vi "Manual.vi"(6 "Cluster":T12={"VISA resource name"="", "baud rate "=115200}, 7 "vi reference":refnum<vi>, 8 "error in (no error)":errorcluster, 9 "IOList_280":T1, 11 "Manual":T4(tab)) -> (0 "error out":errorcluster, 3 "Out reference":refnum<vi>)   [LabVIEW 2015]
uses:
  Control Button/Exit.ctl
  Control Button/Scanner config.ctl
  Control Button/Save.ctl
  Galobal variable_TI.vi
  <vilib>/addons/database/Connection.llb/DB Tools Open Connec (String).vi
  <vilib>/Instr/_visa.llb/VISA Configure Serial Port (Instr).vi
  <vilib>/addons/database/_DB Variant To Data/Database Variant To Data.xnode
  <vilib>/addons/database/NI_Database_API.lvlib
panel:
  out "Array":string[](array[string])
  out "Byte Lenth":i32
  out "error out 2":errorcluster
  in  "Stop":T2
  out "NewVal":T3
  in  "Digital Output":T5
  out "LVDT":string
  out "Digital Input":T6
  in  "Trigger For Model":bool
  in  "Program List":string(combo)
  in  "Home Calling M1":bool
  in  "Stop M1":bool
  in  "SERVO ON CMD M1":bool
  in  "Speed (mm/s) M1":i32=10
  in  "Travel (mm)M1":i32=5
  out "STM1 Done Bit":bool
  out "Error Message":string
  in  "Save":T7
  in  "Sensor Setting Data":T8 {"IL Sensor_Max (AI12)" format="%0.02f"; "IL Sensor_Max (AI11)" format="%0.02f"; "IL Sensor_Max (AI10)" format="%0.02f"; "IL Sensor_Max (AI9)" format="%0.02f"; "IL Sensor1_Max AI1" format="%0.02f"; "IL Sensor1_Max AI0" format="%0.02f"; "IL Sensor_Min (AI12" format="%0.02f"; "IL Sensor_Min (AI11)" format="%0.02f"; "IL Sensor_Min(AI10)" format="%0.02f"; "IL Sensor_Min  (AI9)" format="%0.02f"; "IL Sensor1_ Min AI1" format="%0.02f"; "IL Sensor1_Min AI0" format="%0.02f"}
  out "Sensor Data":T9 {"IL Sensor  (AI12" format="%0.02f"; "IL Sensor (AI11)" format="%0.02f"; "IL Sensor  (AI10)" format="%0.02f"; "IL Sensor (AI9)" format="%0.02f"; "IL Sensor1_AI1" format="%0.02f"; "IL Sensor1_AI0" format="%0.02f"}
  in  "Barcode Trigger":T10(ring)
  out "Error Status":bool
  in  "Scanner config":T11
  out "Read data":string
  out "Boolean":bool
  # "Instruction for Servo motor Operate\n(1)  Switch  ON -OFF  of Fixture Slide servo Brake ON Cmd (P0.19)  \n      from Digital Output tab.\n(2) Switch  ON -OFF  of Fixture Slide Servo Direction Command (P0.20)\n      from Digital Output tab."
  # "Fixture Slide servo"
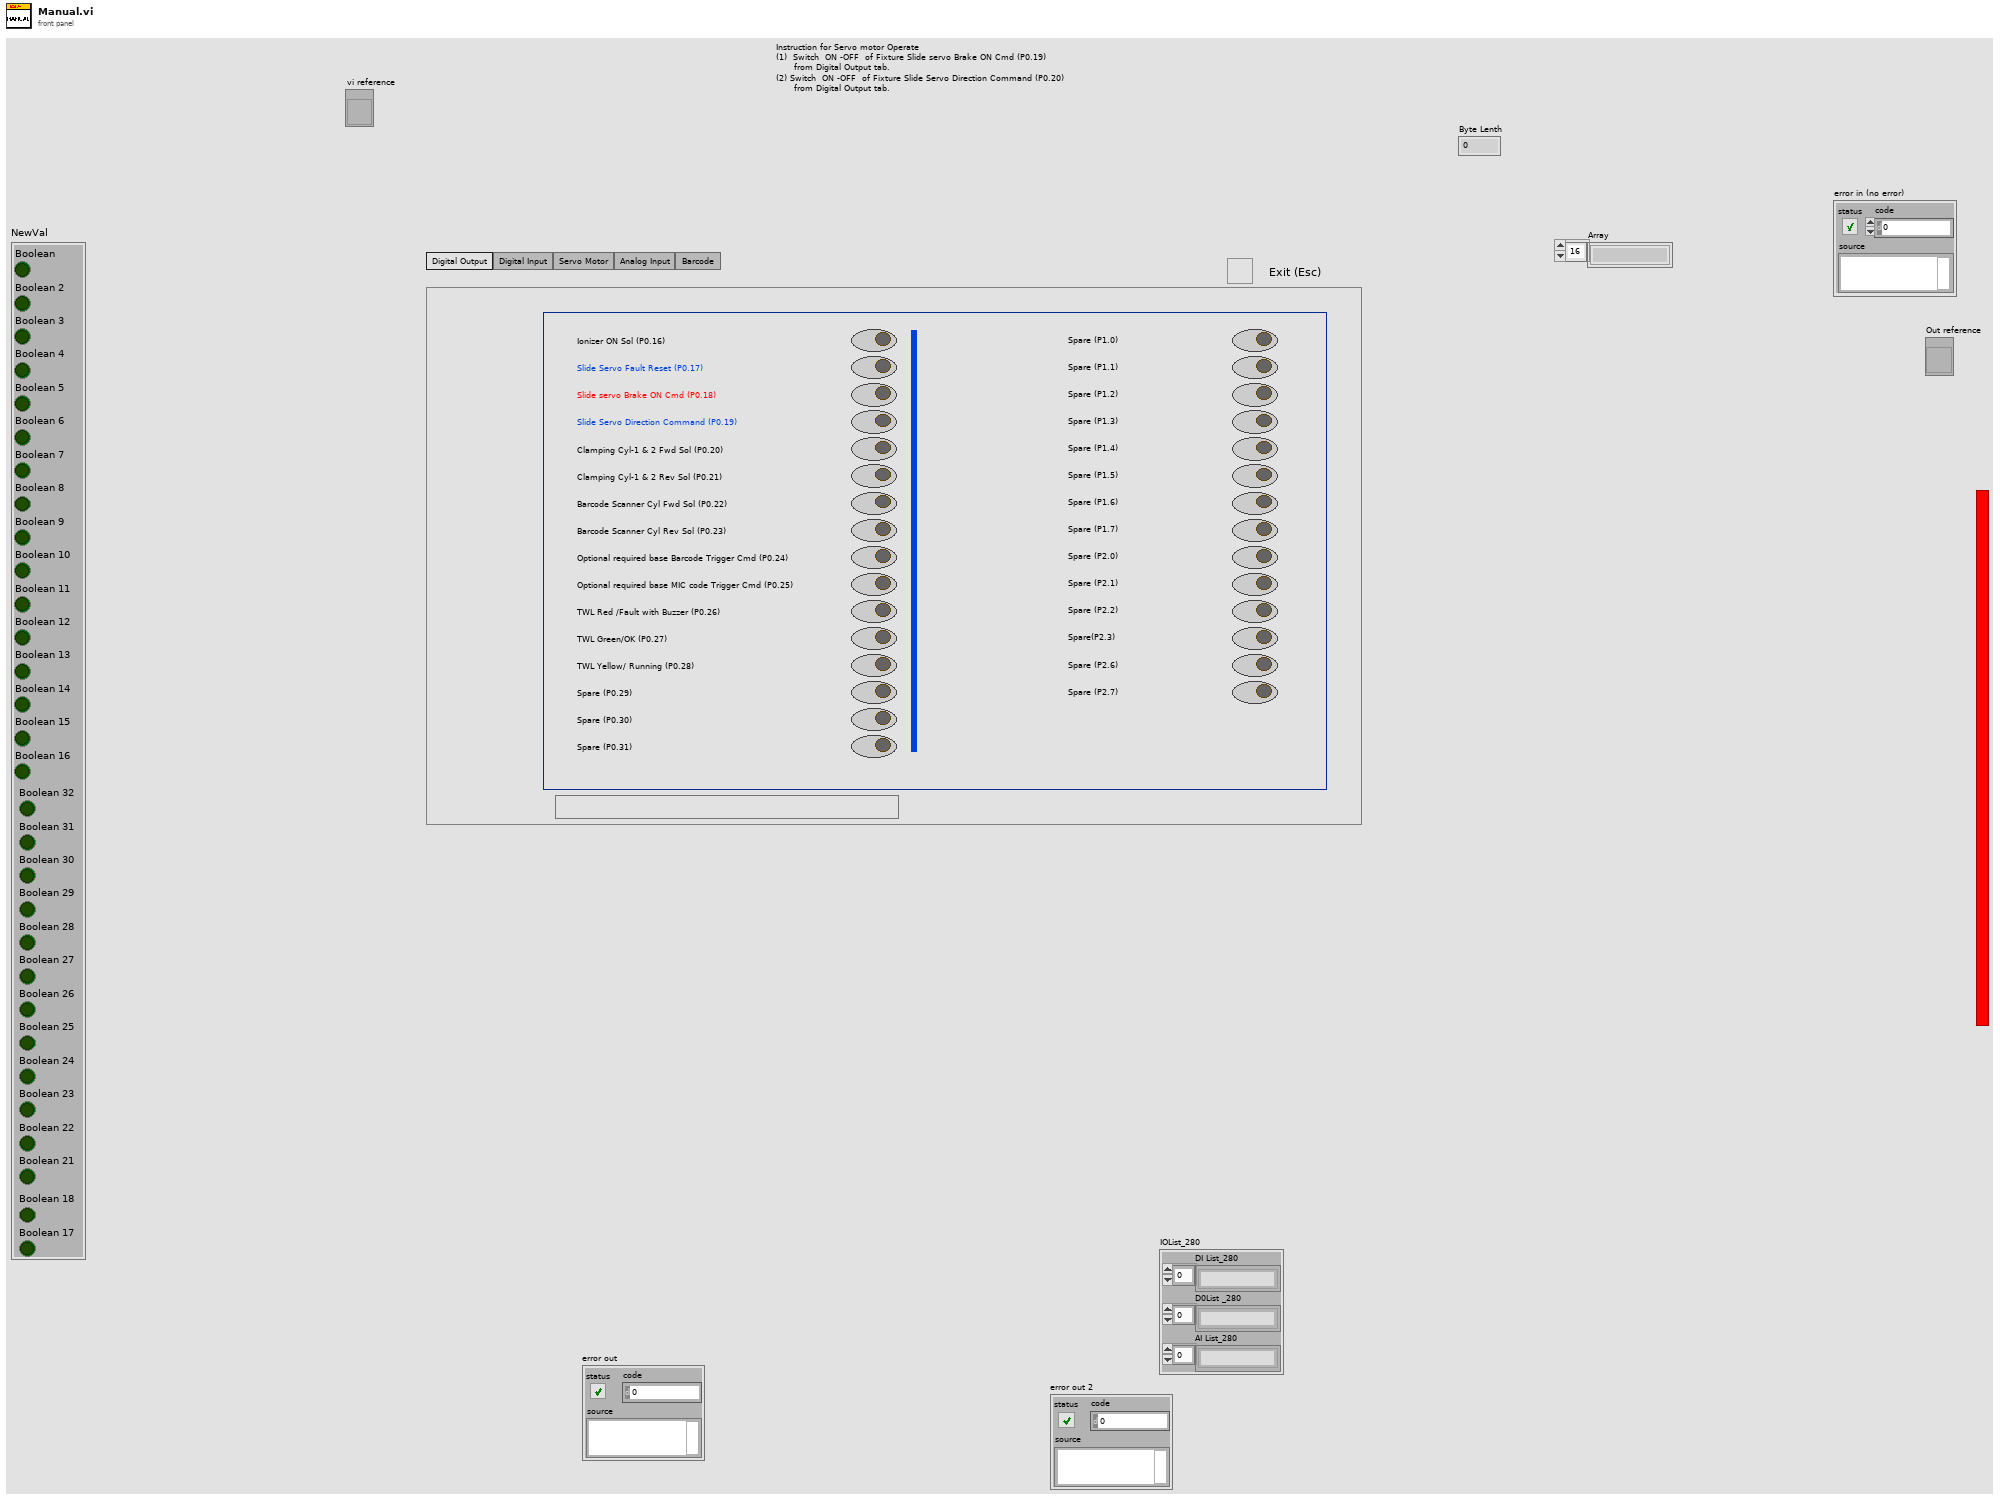
[diagram p1: front panel]
types:
  T1 = cluster{"DI List_280":string[], "D0List _280":string[], "AI List_280":string[]}
  T2 = typedef "Exit.ctl" = bool
  T3 = cluster{"Boolean":bool, "Boolean 2":bool, "Boolean 3":bool, "Boolean 4":bool, "Boolean 5":bool, "Boolean 6":bool, "Boolean 7":bool, "Boolean 8":bool, "Boolean 9":bool, "Boolean 10":bool, "Boolean 11":bool, "Boolean 12":bool, "Boolean 13":bool, "Boolean 14":bool, "Boolean 15":bool, "Boolean 16":bool, "Boolean 17":bool, "Boolean 18":bool, "Boolean 21":bool, "Boolean 22":bool, "Boolean 23":bool, "Boolean 24":bool, "Boolean 25":bool, "Boolean 26":bool, "Boolean 27":bool, "Boolean 28":bool, "Boolean 29":bool, "Boolean 30":bool, "Boolean 31":bool, "Boolean 32":bool}
  T4 = enum32{"Digital Output", "Digital Input", "Servo Motor ", "Analog Input", "Barcode "}
  T5 = cluster{"DO.00":bool, "DO.01":bool, "DO.02":bool, "DO.03":bool, "DO.04":bool, "DO.05":bool, "DO.06":bool, "DO.06":bool, "DO.07":bool, "DO.08":bool, "DO.09":bool, "DO.10":bool, "DO.11":bool, "DO.12":bool, "DO.13":bool, "DO.14":bool, "DO.07 2":bool, "DO.08 2":bool, "DO.09 2":bool, "DO.10 2":bool, "DO.11 2":bool, "DO.12 2":bool, "DO.13 2":bool, "DO.14 2":bool, "DO.00 2":bool, "DO.01 2":bool, "DO.02 2":bool, "DO.03 2":bool, "DO.06 2":bool, "DO.06 3":bool}
  T6 = cluster{"Digital Input":bool, "Digital Input 2":bool, "Digital Input 3":bool, "Digital Input 4":bool, "Digital Input 5":bool, "Digital Input 6":bool, "Digital Input 7":bool, "Digital Input 8":bool, "Digital Input 9":bool, "Digital Input 10":bool, "Digital Input 11":bool, "Digital Input 12":bool, "Digital Input 13":bool, "Digital Input 14":bool, "Digital Input 15":bool, "Digital Input 16":bool, "Digital Input 17":bool, "Digital Input 18":bool, "Digital Input 19":bool, "Digital Input 20":bool, "Digital Input 21":bool, "Digital Input 22":bool, "Digital Input 23":bool, "Digital Input 24":bool, "Digital Input 25":bool, "Digital Input 26":bool, "Digital Input 27":bool, "Digital Input 28":bool, "Digital Input 29":bool, "Digital Input 30":bool, "Digital Input 31":bool, "Digital Input 32":bool, "Digital Input 33":bool, "Digital Input 34":bool, "Digital Input 35":bool, "Digital Input 36":bool, "Digital Input 37":bool, "Digital Input 38":bool, "Digital Input 39":bool, "Digital Input 40":bool, "Digital Input 41":bool, "Digital Input 42":bool, "Digital Input 43":bool, "Digital Input 44":bool}
  T7 = typedef "Save.ctl" = bool
  T8 = cluster{"IL Sensor1_Max AI0":dbl, "IL Sensor1_Min AI0":dbl, "IL Sensor1_Max AI1":dbl, "IL Sensor1_ Min AI1":dbl, "IL Sensor_Max (AI9)":dbl, "IL Sensor_Min  (AI9)":dbl, "IL Sensor_Max (AI10)":dbl, "IL Sensor_Min(AI10)":dbl, "IL Sensor_Max (AI11)":dbl, "IL Sensor_Min (AI11)":dbl, "IL Sensor_Max (AI12)":dbl, "IL Sensor_Min (AI12":dbl}
  T9 = cluster{"IL Sensor1_AI0":dbl, "IL Sensor1_AI1":dbl, "IL Sensor (AI9)":dbl, "IL Sensor  (AI10)":dbl, "IL Sensor (AI11)":dbl, "IL Sensor  (AI12":dbl, "IL Sensor1_AI0":bool, "IL Sensor1_AI1":bool, "IL Sensor1_AI9":bool, "IL Sensor1_AI10":bool, "IL Sensor1_AI11":bool, "IL Sensor1_AI12":bool}
  T10 = enum16{"LCD BArcode Trigger", "MIC Barcode Trigger"}
  T11 = typedef "Scanner config.ctl" = bool
  T12 = cluster{"VISA resource name":refnum<visa-resource-name>, "baud rate ":u32}
  T13 = typedef "NI_Database_API.lvlib/Conn ObjectReference.ctl" = refnum<k1>
  T14 = cluster{" Fixture Brack on":refnum<vi>, " Fixture Direction":refnum<vi>, "Servo Cmd":refnum<vi>, "Servo Home":refnum<vi>}
  T15 = cluster{"Emergency_1":bool, "Reset_2":bool, "Air Pressure_4":bool, "Safety Sensor_5":bool, "Safety Sensor_6":bool, "Barcode Rev rs_24":bool, "Clamp fwd rs_21":bool, "Servo Fault":bool, "Home _3":bool}
  T16 = cluster{"IL Sensor1_AI0":dbl, "IL Sensor1_AI1":dbl, "IL Sensor (AI6)":dbl, "IL Sensor  (AI7)":dbl, "IL Sensor (AI8)":dbl, "IL Sensor  (AI9)":dbl, "IL Sensor1_AI0":bool, "IL Sensor1_AI1":bool, "IL Sensor1_AI9":bool, "IL Sensor1_AI10":bool, "IL Sensor1_AI11":bool, "IL Sensor1_AI12":bool}
  T17 = cluster{"Digital input[0]":bool, "Digital input[1]":bool, "Digital input[2]":bool, "Digital input[3]":bool, "Digital input[4]":bool, "Digital input[5]":bool, "Digital input[6]":bool, "Digital input[7]":bool, "Digital input[8]":bool, "Digital input[9]":bool, "Digital input[10]":bool, "Digital input[11]":bool, "Digital input[12]":bool, "Digital input[13]":bool, "Digital input[14]":bool, "Digital input[15]":bool, "Digital input[16]":bool, "Digital input[17]":bool, "Digital input[18]":bool, "Digital input[19]":bool, "Digital input[20]":bool, "Digital input[21]":bool, "Digital input[22]":bool, "Digital input[23]":bool, "Digital input[24]":bool, "Digital input[25]":bool, "Digital input[26]":bool, "Digital input[27]":bool, "Digital input[28]":bool, "Digital input[29]":bool, "Digital input[30]":bool, "Digital input[31]":bool, "Digital input[32]":bool, "Digital input[33]":bool, "Digital input[34]":bool, "Digital input[35]":bool, "Digital input[36]":bool, "Digital input[37]":bool, "Digital input[38]":bool, "Digital input[39]":bool, "Digital input[40]":bool, "Digital input[41]":bool, "Digital input[42]":bool, "Digital input[43]":bool}
  T18 = cluster{"IL Sensor1_Max AI0":dbl, "IL Sensor1_Min AI0":dbl, "IL Sensor1_Max AI1":dbl, "IL Sensor1_ Min AI1":dbl, "IL Sensor_Max (AI9)":dbl, "IL Sensor_Min  (AI9)":dbl, "IL Sensor_Max (AI10)":dbl, "IL Sensor_Min(AI10)":dbl, "IL Sensor_Max (AI11)":dbl, "IL Sensor_Min (AI11)":dbl, "IL Sensor_Max (AI12)":dbl, "IL Sensor_Min (AI12":dbl, "Key":string}
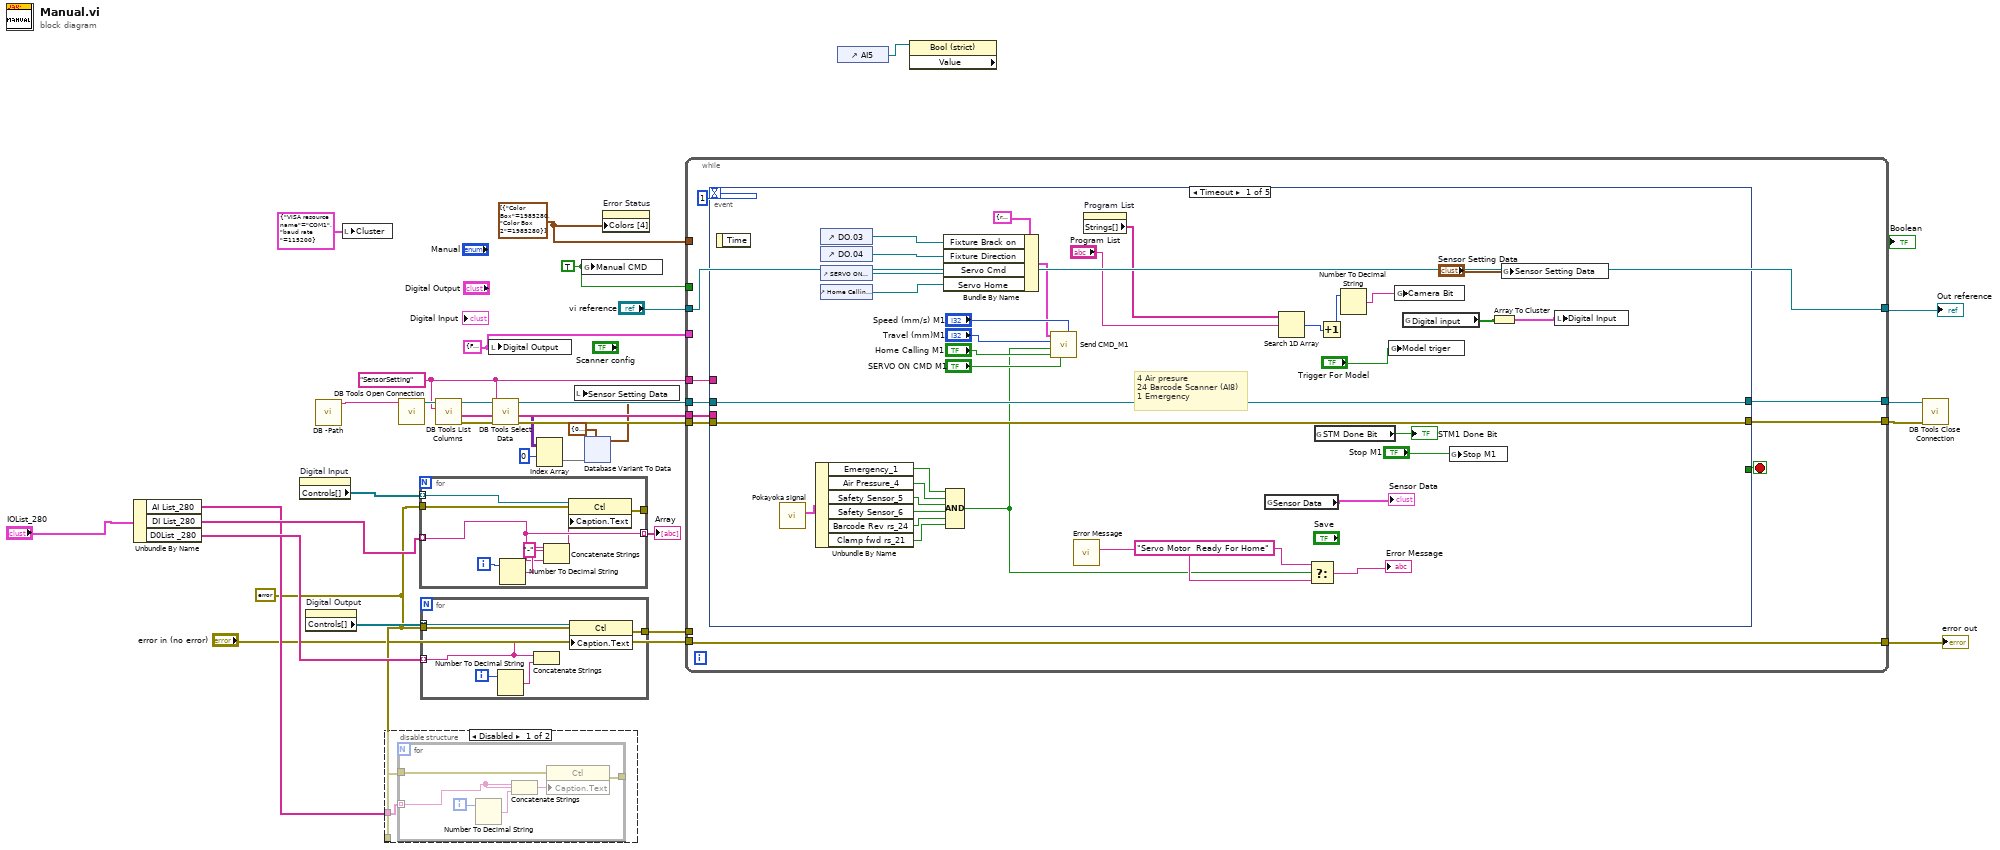
[diagram p0: block diagram]
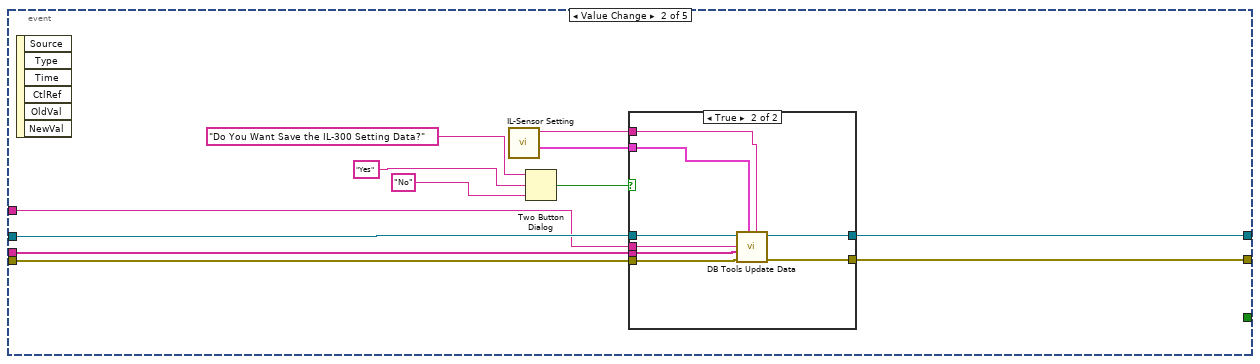
[diagram p3: hidden frame]
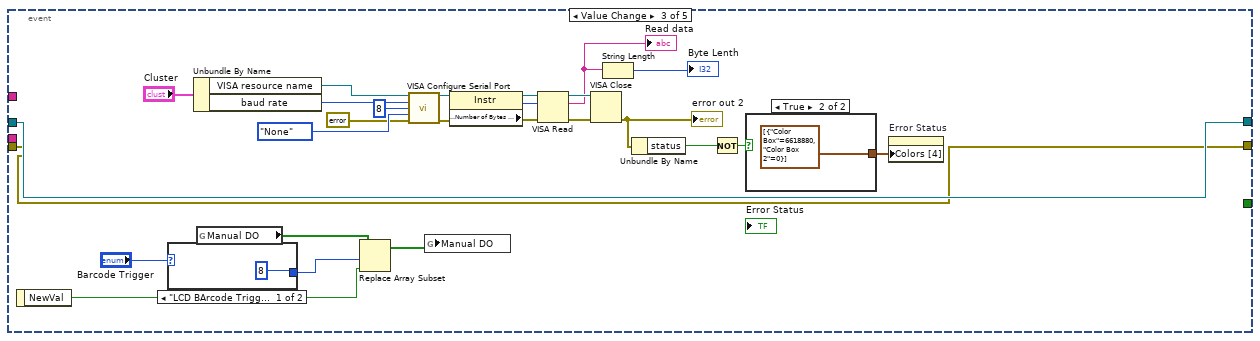
[diagram p5: hidden frame]
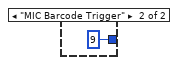
[diagram p6: hidden frame]
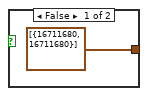
[diagram p7: hidden frame]
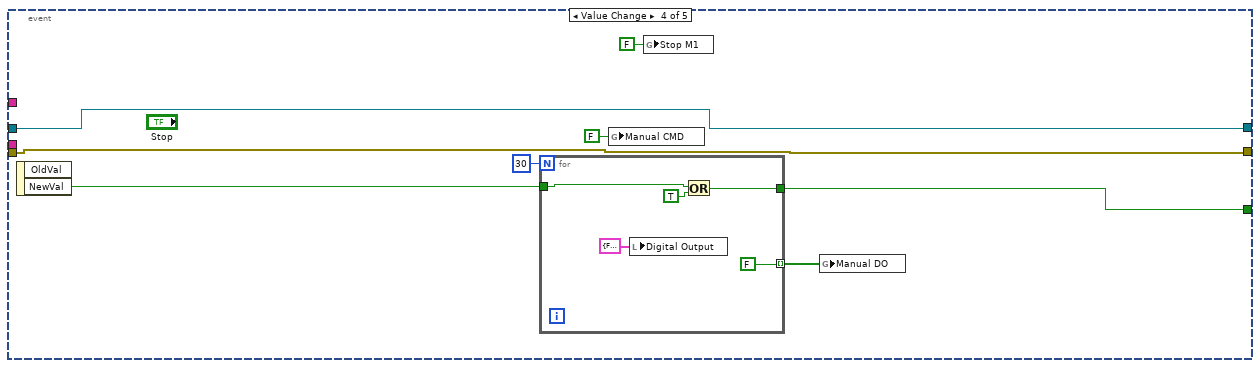
[diagram p8: hidden frame]
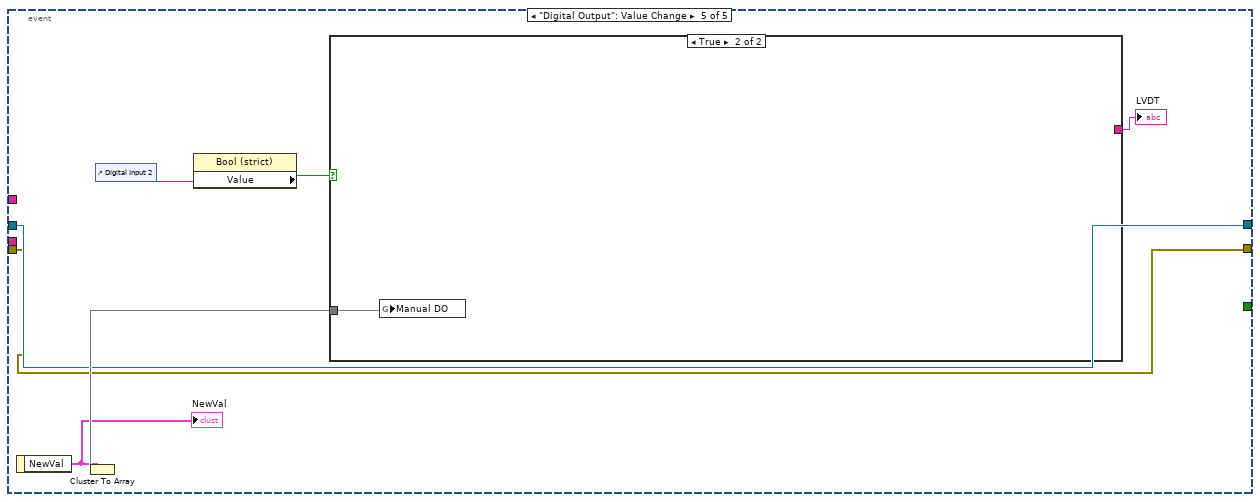
[diagram p9: hidden frame]
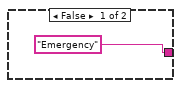
[diagram p10: hidden frame]
diagram:
  w11 = "SensorSetting" ("table")
  w18 = T5 {"DO.00"=FALSE, "DO.01"=FALSE, "DO.02"=FALSE, "DO.03"=FALSE, "DO.04"=FALSE, "DO.05"=FALSE, "DO.06"=FALSE, "DO.06"=FALSE, "DO.07"=FALSE, "DO.08"=FALSE, "DO.09"=FALSE, "DO.10"=FALSE, "DO.11"=FALSE, "DO.12"=FALSE, "DO.13"=FALSE, "DO.14"=FALSE, "DO.07 2"=FALSE, "DO.08 2"=FALSE, "DO.09 2"=FALSE, "DO.10 2"=FALSE, "DO.11 2"=FALSE, "DO.12 2"=FALSE, "DO.13 2"=FALSE, "DO.14 2"=FALSE, "DO.00 2"=FALSE, "DO.01 2"=FALSE, "DO.02 2"=FALSE, "DO.03 2"=FALSE, "DO.06 2"=FALSE, "DO.06 3"=FALSE} ("Digital Output")
  w21 = errorcluster {"status"=FALSE, "code"=0, "source"=""} ("error in (no error)")
  w24 = cluster{"Color Box":u32, "Color Box 2":u32}[] [{"Color Box"=1985280, "Color Box 2"=1985280}] ("Colors [4]")
  w29 = TRUE ("Manual CMD")
  n1 = Unbundle By Name("IOList_280") -> ("AI List_280"=w25:string[], "DI List_280"=w26:string[], "D0List _280"=w28:string[])
  n2 = property on="Digital Input" class="Clust (strict)"() -> ("Controls[]"=w27:refnum<vi>[])  [unwired: 2 in, 2 out]
  n3 = property on="Digital Output" class="Clust (strict)"() -> ("Controls[]"=w32:refnum<vi>[])  [unwired: 2 in, 2 out]
  n4 = call "DB -Path.vi"() -> ("String"=w15:string)  [unwired: 11 in]
  n5 = local write "Cluster"(T12 {"VISA resource name"="COM1", "baud rate "=115200} ("Cluster")) -> ()
  n6 = disable-structure shown="Disabled" {
    disable-tunnel: w25 -> [w35 _]
    disable-tunnel: w21 -> [w34 _]
    frame Disabled {
      n7 = for {
        tunnel: [w39] -> _
        tunnel: w34 -> [w37]
        tunnel: w35 -> [w36] mode=indexing
        i -> [w40]
        n8 = Number To Decimal String(number=w40) -> (decimal integer string=w38:string)  [unwired: 1 in]
        n9 = Concatenate Strings(w36, w38) -> ()  [unwired: 1 out]
        n10 = property class="Ctl"(error in=w37, "Caption.Text"=w36) -> (error out=w39:errorcluster)  [unwired: 1 in, 1 out]
      }
    }
    frame Enabled {
    }
  }
  n11 = call-poly <vilib>:"DB Tools Open Connection.vi"("connection information"=w15) -> ("connection reference"=w16:T13)  [unwired: 7 in, 1 out]
  n12 = for {
    tunnel: w27 -> [w48] mode=indexing
    tunnel: [w46] -> _
    tunnel: w21 -> [w45]
    tunnel: w26 -> [w42] mode=indexing
    tunnel: [w42] -> w22 mode=indexing
    i -> [w47]
    n13 = Number To Decimal String(number=w47) -> (decimal integer string=w44:string)  [unwired: 1 in]
    n14 = Concatenate Strings(w44, "-" ("string"), w42) -> (w41:string)
    n15 = property class="Ctl"(reference=w48, error in=w45, "Caption.Text"=w41) -> (error out=w46:errorcluster)  [unwired: 1 out]
  }
  "Array" <- w22
  n16 = for {
    tunnel: w32 -> [w54] mode=indexing
    tunnel: [w52] -> w33
    tunnel: w21 -> [w50]
    tunnel: w28 -> [w49] mode=indexing
    i -> [w53]
    n17 = Number To Decimal String(number=w53) -> (decimal integer string=w51:string)  [unwired: 1 in]
    n18 = Concatenate Strings(w49, w51) -> ()  [unwired: 1 out]
    n19 = property class="Ctl"(reference=w54, error in=w50, "Caption.Text"=w49) -> (error out=w52:errorcluster)  [unwired: 1 out]
  }
  n20 = call <vilib>:"DB Tools List Columns.vi"("table"=w11, "connection reference"=w16) -> ("error out"=w8:errorcluster, "columns"=w12:string[], "connection reference out"=w10:T13)  [unwired: 2 in, 1 out]
  n21 = local write "Digital Output"(w18) -> ()
  n22 = call <vilib>:"DB Tools Select Data.vi"("error in (no error)"=w8, "columns"=w12, "table"=w11, "connection reference"=w10) -> ("error out"=w7:errorcluster, "data"=w3:variant[][], "connection reference out"=w9:T13)  [unwired: 2 in]
  n23 = Index Array(array=w3, index (row)=0) -> (element=w5:variant[])  [unwired: 1 in]
  n24 = global write "Galobal variable_TI.vi" "Manual CMD"(w29) -> ()
  n25 = xnode "Database Variant To Data"("database variant"=w5, "type"=T8 {"IL Sensor1_Max AI0"=0.0, "IL Sensor1_Min AI0"=0.0, "IL Sensor1_Max AI1"=0.0, "IL Sensor1_ Min AI1"=0.0, "IL Sensor_Max (AI9)"=0.0, "IL Sensor_Min  (AI9)"=0.0, "IL Sensor_Max (AI10)"=0.0, "IL Sensor_Min(AI10)"=0.0, "IL Sensor_Max (AI11)"=0.0, "IL Sensor_Min (AI11)"=0.0, "IL Sensor_Max (AI12)"=0.0, "IL Sensor_Min (AI12"=0.0} ("Sensor Setting Data")) -> ("data"=w2:T8)  [unwired: 1 in, 1 out]
  n26 = local write "Sensor Setting Data"(w2) -> ()
  n27 = property on="Error Status" class="Bool (strict)"("Colors [4]"=w24) -> ()  [unwired: 2 in, 2 out]
  n28 = while {
    tunnel: w33 -> [_]
    tunnel: [w62] -> w31
    tunnel: "vi reference" -> [w63]
    tunnel: [w63] -> w30
    tunnel: w29 -> [_]
    tunnel: w24 -> [_]
    tunnel: "error in (no error)" -> [w62]
    tunnel: w18 -> [_]
    tunnel: w9 -> [w60]
    tunnel: w7 -> [w59]
    tunnel: w12 -> [w58]
    tunnel: w11 -> [w57]
    tunnel: [w56] -> w14
    tunnel: [w55] -> w13
    stop <- w61 stop-if-true
    n29 = event shown="[0] Timeout" {
      selector: _ -> [_ _ _ _ _]
      dyn-events: _ -> [_ _ _ _ _]
      timeout: 1 -> [_ _ _ _ _]
      tunnel: [_ _ _ w154 _] -> w61
      tunnel: w60 -> [w80 w111 w128 w153 w168]
      tunnel: w59 -> [w79 w110 w127 w152 w167]
      tunnel: w58 -> [_ w109 _ _ _]
      tunnel: w57 -> [_ w108 _ _ _]
      tunnel: [w80 w107 w128 w153 w168] -> w56
      tunnel: [w79 w106 w127 w152 w167] -> w55
      event Timeout {
        # "4 Air presure\n24 Barcode Scanner (AI8)\n1 Emergency"
        n30 = event-data() -> ()  [unwired: 1 in, 1 out]
        n31 = call "Pokayoka signal.vi"() -> ("output cluster"=w78:T15)  [unwired: 10 in, 1 out]
        n32 = Unbundle By Name(w78) -> ("Emergency_1"=w72:bool, "Air Pressure_4"=w71:bool, "Safety Sensor_5"=w77:bool, "Safety Sensor_6"=w76:bool, "Barcode Rev rs_24"=w75:bool, "Clamp fwd rs_21"=w74:bool)
        n33 = control-ref of="DO.03"() -> (w92:refnum<vi>)
        n34 = control-ref of="DO.04"() -> (w91:refnum<vi>)
        n35 = control-ref of="SERVO ON CMD M1"() -> (w89:refnum<vi>)
        n36 = control-ref of="Home Calling M1"() -> (w90:refnum<vi>)
        n37 = Bundle By Name(cluster=T14 {" Fixture Brack on"=refnum, " Fixture Direction"=refnum, "Servo Cmd"=refnum, "Servo Home"=refnum} ("Slide Servo"), "Fixture Brack on"=w92, "Fixture Direction"=w91, "Servo Cmd"=w89, "Servo Home"=w90) -> (w88:T14)
        n38 = Compound Arithmetic op=AND(w72, w71, w77, w76, w75, w74) -> (w73:bool)
        n39 = call "Send CMD_M1.vi"("Speed (mm/s) M1"="Speed (mm/s) M1", "SERVO ON CMD M1"="SERVO ON CMD M1", "Home Calling M1"="Home Calling M1", "Pokayoka"=w73, "Travel (mm)M1"="Travel (mm)M1", "Slide Servo"=w88) -> ()  [unwired: 6 in]
        n40 = call "Error Message.vi"() -> ("Error"=w84:string)  [unwired: 11 in]
        n41 = property on="Program List" class="CmbBox"() -> ("Strings[]"=w69:string[])  [unwired: 2 in, 2 out]
        n42 = global read "Galobal variable_TI.vi" "Sensor Data"() -> (→"Sensor Data":T16)
        n43 = Search 1D Array(1D array=w69, element="Program List") -> (index of element=w70:i32)  [unwired: 1 in]
        n44 = Select(t="Servo Motor  Ready For Home", s=w73, f=w84) -> (s? t:f=→"Error Message":string)
        n45 = global read "Galobal variable_TI.vi" "STM Done Bit"() -> (→"STM1 Done Bit":bool)
        n46 = Increment(x=w70) -> (x+1=w67:i32)
        n47 = Number To Decimal String(number=w67) -> (decimal integer string=w66:string)  [unwired: 1 in]
        n48 = global write "Galobal variable_TI.vi" "Model triger"("Trigger For Model") -> ()
        n49 = global write "Galobal variable_TI.vi" "Camera Bit"(w66) -> ()
        n50 = global read "Galobal variable_TI.vi" "Digital input"() -> (w87:bool[])
        n51 = global write "Galobal variable_TI.vi" "Stop M1"("Stop M1") -> ()
        n52 = Array To Cluster(array=w87) -> (cluster=w99:T17)
        n53 = global write "Galobal variable_TI.vi" "Sensor Setting Data"("Sensor Setting Data") -> ()
        n54 = local write "Digital Input"(w99) -> ()
      }
      event Value Change {
        n55 = event-data() -> ()  [unwired: 1 in, 6 out]
        n56 = call "IL-Sensor Setting.vi"() -> ("IL Sensor"=w104:T18, "Search Key"=w105:string)  [unwired: 10 in]
        n57 = Two Button Dialog(message="Do You Want Save the IL-300 Setting Data?", 1:"No" ("F button name (\"Cancel\")"), 2:"Yes" ("T button name (\"OK\")")) -> (T button?=w103:bool)
        n58 = case shown="True" w103 {
          tunnel: w111 -> [w113 w121]
          tunnel: w110 -> [w112 w120]
          tunnel: w109 -> [_ w119]
          tunnel: w108 -> [_ w118]
          tunnel: [w113 w117] -> w107
          tunnel: [w112 w116] -> w106
          tunnel: w105 -> [_ w115]
          tunnel: w104 -> [_ w114]
          frame False {
          }
          frame True {
            n59 = call <vilib>:"DB Tools Update Data.vi"("condition"=w115, "data"=w114, "error in (no error)"=w120, "columns"=w119, "table"=w118, "connection reference"=w121) -> ("error out"=w116:errorcluster, "connection reference out"=w117:T13)  [unwired: 4 in]
          }
        }
      }
      event Value Change {
        n60 = event-data() -> ("NewVal"=w124:T11)  [unwired: 1 in]
        n61 = case shown="\"LCD BArcode Trigger\", Default" "Barcode Trigger" {
          tunnel: [8 ("index") 9 ("index")] -> w122
          frame "LCD BArcode Trigger", Default {
          }
          frame "MIC Barcode Trigger" {
          }
        }
        n62 = Unbundle By Name("Cluster") -> ("VISA resource name"=w147:refnum<visa-resource-name>, "baud rate"=w146:u32)
        n63 = global read "Galobal variable_TI.vi" "Manual DO"() -> (w125:bool[])
        n64 = Replace Array Subset(array=w125, new element=w124, index=w122) -> (w126:bool[])
        n65 = call-poly "VISA Configure Serial Port"("VISA resource name"=w147, "baud rate (9600)"=w146, "data bits (8)"=u16 8, "parity (0:none)"=enum16{"None", "Odd", "Even", "Mark", "Space"}."None", "error in (no error)"=errorcluster {"status"=FALSE, "code"=0, "source"=""} ("error in (no error) 2")) -> ("VISA resource name out"=w145:refnum<visa-resource-name>, "error out"=w143:errorcluster)  [unwired: 9 in]
        n66 = global write "Galobal variable_TI.vi" "Manual DO"(w126) -> ()
        n67 = property class="Instr"(reference=w145, error in=w143) -> (reference out=w144:refnum<visa-resource-name>, error out=w142:errorcluster, "Serial Settings:Number of Bytes at Serial Port"=w141:u32)
        n68 = VISA Read(VISA resource name=w144, byte count=w141, error in (no error)=w142) -> (VISA resource name out=w139:refnum<visa-resource-name>, read buffer=w137:string, error out=w138:errorcluster)  [unwired: 1 out]
        "Read data" <- w137
        n69 = VISA Close(VISA resource name=w139, error in (no error)=w138) -> (error out=w135:errorcluster)
        "error out 2" <- w135
        n70 = String Length(string=w137) -> (length=→"Byte Lenth":i32)
        n71 = Unbundle By Name(w135) -> ("status"=w134:bool)
        n72 = Not(x=w134) -> (.not. x?=w132:bool)
        n73 = case shown="True" w132 {
          tunnel: [cluster{"Color Box":u32, "Color Box 2":u32}[] [{"Color Box"=16711680, "Color Box 2"=16711680}] ("Colors [4]") cluster{"Color Box":u32, "Color Box 2":u32}[] [{"Color Box"=6618880, "Color Box 2"=0}] ("Colors [4]")] -> w133
          frame False {
          }
          frame True {
          }
        }
        n74 = property on="Error Status" class="Bool (strict)"("Colors [4]"=w133) -> ()  [unwired: 2 in, 2 out]
      }
      event Value Change {
        n75 = event-data() -> ("NewVal"=w155:T2)  [unwired: 1 in, 1 out]
        n76 = for {
          N: 30 -> [_]
          tunnel: [FALSE] -> w157 mode=indexing
          tunnel: w155 -> [w162]
          tunnel: [w161] -> w154
          n77 = local write "Digital Output"(T5 {"DO.00"=FALSE, "DO.01"=FALSE, "DO.02"=FALSE, "DO.03"=FALSE, "DO.04"=FALSE, "DO.05"=FALSE, "DO.06"=FALSE, "DO.06"=FALSE, "DO.07"=FALSE, "DO.08"=FALSE, "DO.09"=FALSE, "DO.10"=FALSE, "DO.11"=FALSE, "DO.12"=FALSE, "DO.13"=FALSE, "DO.14"=FALSE, "DO.07 2"=FALSE, "DO.08 2"=FALSE, "DO.09 2"=FALSE, "DO.10 2"=FALSE, "DO.11 2"=FALSE, "DO.12 2"=FALSE, "DO.13 2"=FALSE, "DO.14 2"=FALSE, "DO.00 2"=FALSE, "DO.01 2"=FALSE, "DO.02 2"=FALSE, "DO.03 2"=FALSE, "DO.06 2"=FALSE, "DO.06 3"=FALSE} ("Digital Output")) -> ()
          n78 = Or(x=w162, y=TRUE) -> (x .or. y?=w161:T2)
        }
        n79 = global write "Galobal variable_TI.vi" "Manual CMD"(FALSE ("Manual CMD")) -> ()
        n80 = global write "Galobal variable_TI.vi" "Stop M1"(FALSE ("Stop M1")) -> ()
        n81 = global write "Galobal variable_TI.vi" "Manual DO"(w157) -> ()
      }
      event "Digital Output": Value Change {
        n82 = event-data() -> ("NewVal"=w169:T5)  [unwired: 1 in]
        "NewVal" <- w169
        n83 = Cluster To Array(cluster=w169) -> (array=w170:bool[])
        n84 = control-ref of="Digital Input 2"() -> (w166:refnum<vi>)
        n85 = property class="Bool (strict)"(reference=w166) -> ("Value"=w165:bool)  [unwired: 1 in, 2 out]
        n86 = case shown="True" w165 {
          tunnel: ["Emergency" _] -> w171
          tunnel: w170 -> [_ w173]
          frame False {
          }
          frame True {
            n87 = global write "Galobal variable_TI.vi" "Manual DO"(w173) -> ()
          }
        }
        "LVDT" <- w171
      }
    }
  }
  "error out" <- w31
  "Out reference" <- w30
  n88 = control-ref of="AI5"() -> (w17:refnum<vi>)
  n89 = property class="Bool (strict)" props=["Value"](reference=w17) -> ()  [unwired: 1 in, 3 out]
  n90 = call <vilib>:"DB Tools Close Connection.vi"("error in (no error)"=w13, "connection reference"=w14) -> ()  [unwired: 5 in, 1 out]
